vi "Do Action.vi"(4 "error in (no error)":errorcluster, 6 "Array in":refnum<class>[](array[class]), 7 "Act_Set One in":refnum<class "Act_Set One.lvclass">) -> (0 "error out":errorcluster, 2 "Array out":refnum<class>[](array[class]), 3 "Act_Set One out":refnum<class "Act_Set One.lvclass">)   [LabVIEW 2014, in "Act_Set One.lvclass"]
uses:
  Act_Set One.lvclass
  Act_Set One.lvclass/Act_Set One.ctl
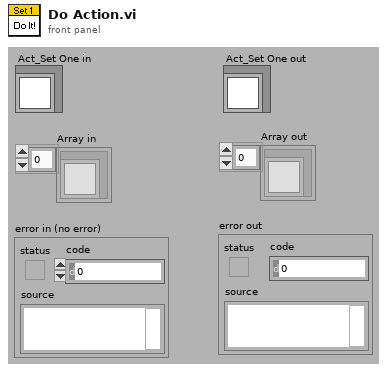
[diagram p1: front panel]
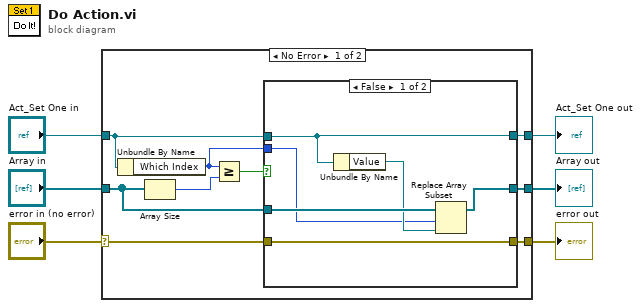
[diagram p0: block diagram]
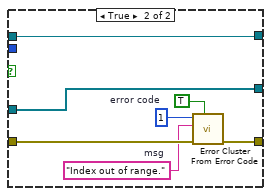
[diagram p2: hidden frame]
diagram:
  n1 = case shown="No Error" "error in (no error)" {
    selector: "error in (no error)" -> [w13 w31]
    tunnel: [w12 w31] -> w5
    tunnel: "Array in" -> [w11 w29]
    tunnel: "Act_Set One in" -> [w10 w30]
    tunnel: [w8 w29] -> w2
    tunnel: [w7 w30] -> w1
    frame No Error {
      n2 = Unbundle By Name(w10) -> ("Which Index"=w9:i32)
      n3 = Array Size(array=w11) -> (size(s)=w15:i32)
      n4 = Greater Or Equal?(x=w9, y=w15) -> (x >= y?=w14:bool)
      n5 = case shown="False" w14 {
        tunnel: w13 -> [w16 w28]
        tunnel: [w16 w27] -> w12
        tunnel: w11 -> [w21 w22]
        tunnel: w10 -> [w17 w23]
        tunnel: w9 -> [w19 _]
        tunnel: [w18 w22] -> w8
        tunnel: [w17 w23] -> w7
        frame False {
          n6 = Unbundle By Name(w17) -> ("Value"=w20:refnum<class>)
          n7 = Replace Array Subset(array=w21, new element=w20, index=w19) -> (w18:refnum<class>[])
        }
        frame True {
          w25 = "Index out of range."  # msg
          w26 = 1  # error code
          n8 = call <vilib>:"Error Cluster From Error Code.vi"("show call chain? (False)"=TRUE ("show call chain?"), "error in (no error)"=w28, "error message (\"\")"=w25, "error code (0)"=w26) -> ("error out"=w27:errorcluster)  [unwired: 5 in]
        }
      }
    }
    frame Error {
    }
  }
  "error out" <- w5
  "Array out" <- w2
  "Act_Set One out" <- w1
